vi "Plot_Space_Analysis.vi"(0 "Table":string[][](table)) -> ()   [LabVIEW 2015]
uses:
  <vilib>/Utility/miscctls.llb/LVRowAndColumnUnsignedTypeDef.ctl
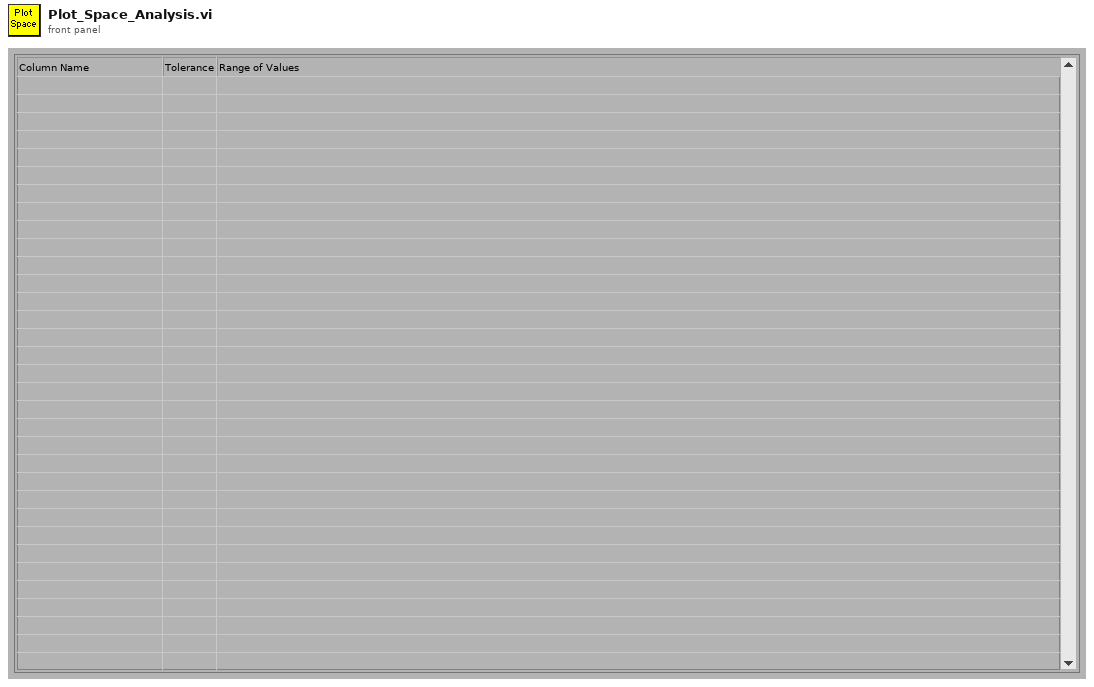
[diagram p1: front panel]
types:
  T1 = typedef "LVRowAndColumnUnsignedTypeDef.ctl" = cluster{"Row":u32, "Column":u32}
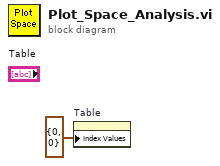
[diagram p0: block diagram]
diagram:
  n1 = property on="Table" class="Tbl (strict)"("Index Values"=T1 {"Row"=0, "Column"=0}) -> ()  [unwired: 2 in, 2 out]
